vi "Running Array Difference.vi"(1 "?":dbl[](array[numeric]) format="%.2e", 2 "?":dbl[](array[numeric]) format="%.2e", 3 "?":dbl[](array[numeric]) format="%.2e", 4 "Point #":i32) -> (0 "?":dbl[](array[numeric]) format="%.2e")   [LabVIEW 2019]
doc: "This VI takes a running difference of 3arrays. The value returned is the average of the 1st and 3rd measurements minus the 2nd measurement over 2.\nScott Hannahs, NHMFL - FSU, April 1995"
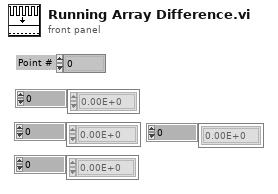
[diagram p1: front panel]
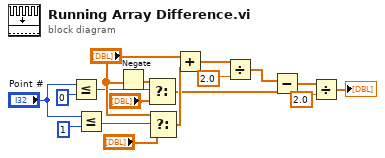
[diagram p0: block diagram]
diagram:
  n1 = Less Or Equal?(x="Point #", y=0) -> (x <= y?=w10:bool)
  n2 = Less Or Equal?(x="Point #", y=1) -> (x <= y?=w7:bool)
  n3 = Negate(x="?") -> (-x=w11:dbl[])
  n4 = Select(t=w11, s=w10, f="?") -> (s? t:f=w13:dbl[])
  n5 = Select(t="?", s=w7, f="?") -> (s? t:f=w14:dbl[])
  n6 = Add(x="?", y=w14) -> (x+y=w15:dbl[])
  n7 = Divide(x=w15, y=2.0) -> (x/y=w17:dbl[])
  n8 = Subtract(x=w17, y=w13) -> (x-y=w2:dbl[])
  n9 = Divide(x=w2, y=2.0) -> (x/y=→"?":dbl[])
